vi "Crop Video Time Utility.vi"() -> ()   [LabVIEW 2017]
uses:
  LabVIEW/Controls/Crop Video State.ctl
  LabVIEW/Controls/Frame Grabber Data.ctl
  <vilib>/userdefined/High Color/IMAQdx.ctl
  <vilib>/vision/Image Controls.llb/IMAQ Image.ctl
  <vilib>/vision/Avi.llb/IMAQ AVI2 Refnum.ctl
  LabVIEW/Controls/Rigid Body Info.ctl
  LabVIEW/Controls/Position.ctl
  LabVIEW/Controls/Orientation.ctl
  LabVIEW/Controls/Refnums.ctl
  LabVIEW/Controls/Dimensions.ctl
  LabVIEW/Controls/Room Dimensions.ctl
panel:
  in  "Help":bool
  in  "Codec":u16(ring) items=["Cinepak Codec by Radius", "Intel IYUV codec", "Microsoft Video 1", "FF Video Codec 1 (FFV1) (NI Vision)", "Motion JPEG (NI Vision)", "Y800 Uncompressed Grey Scale (NI Vision)", "YUV 4:2:0 Planar (NI Vision)"]
  out "Number of Playback Frames":i32
  in  "Crop Inside":bool
  in  "Playback Rate":dbl(knob) min=1.0 max=100.0 scale=1.0..100.0
  in  "Crop Outside":bool
  in  "Play":bool
  in  "Frame Slider":cluster{i32, i32, i32}(slide)={9, 173, 93} scale=0.0..1.0
  out "Saving":bool
  in  "Stop":bool
  out "Video path":path
  in  "Load":bool
  out "Frame":T1(plugin-control)
  # "Frame"
  # "of"
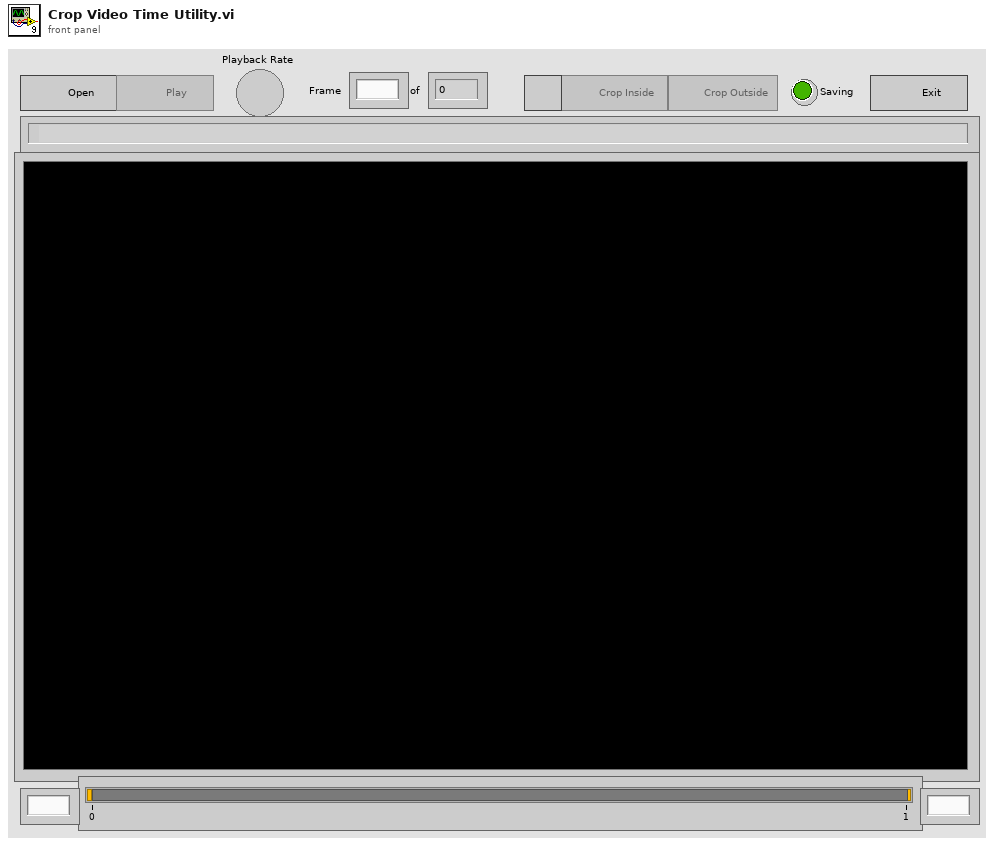
[diagram p1: front panel]
types:
  T1 = typedef "IMAQ Image.ctl" = refnum<image>
  T2 = typedef "Frame Grabber Data.ctl" = cluster{"Camera Session":T3, "Frame":T1, "AVI Refnum":T4, "Codecs":string[], "Frame number":u32, "Tracking File Refnum":refnum<file>, "Tick Count":u32, "Probe Object":refnum<vi>, "Playback Probe Data":dbl[][], "Rigid Body":T5, "Total no frames playback":i32, "Video FPS":dbl, "Camera connected?":bool, "Scene":refnum<vi>, "Cropped Frame":T1, "Tracker FPS":dbl, "Crop ROI":i32[], "Presentation Values":string[], "Elapsed time (ms)":u32, "Camera frames playback":u32, "Refnums":T8, "Dimensions":T9, "Playback Data As Strings":string[][], "Cropped Tracking File Refnum":refnum<file>, "Cropped AVI Refnum":T4, "Header":string[]}
  T3 = typedef "IMAQdx.ctl" = refnum<k21>
  T4 = typedef "IMAQ AVI2 Refnum.ctl" = refnum<k20>
  T5 = typedef "Rigid Body Info.ctl" = cluster{"Position":T6, "Orientation":T7, "Quaternion":cluster{"qx":sgl, "qy":sgl, "qz":sgl, "qw":sgl}, "Tracked?":bool}
  T6 = typedef "Position.ctl" = cluster{"x (mm)":sgl, "y (mm)":sgl, "z (mm)":sgl}
  T7 = typedef "Orientation.ctl" = cluster{"Pitch (rad)":sgl, "Yaw (rad)":sgl, "Roll (rad)":sgl}
  T8 = typedef "Refnums.ctl" = cluster{"Live Refnum":refnum<vi>, "Record Refnum":refnum<vi>, "Recording Settings Refnum":refnum<vi>, "Playback Refnum":refnum<vi>, "Frame Slider Refnum":refnum<vi>, "Pause Refnum":refnum<vi>, "Home Refnum":refnum<vi>, "Crop Refnum":refnum<vi>, "Clear Crop Refnum":refnum<vi>, "stop refnum":refnum<vi>, "Playback Rate Refnum":refnum<vi>, "Operator Settings Refnums":refnum<vi>, "Presentation Refnum":refnum<vi>, "Gestation Refnum":refnum<vi>, "Connection Settings Refnum":refnum<vi>, "Crop Time Frame Slider Refnum":refnum<vi>}
  T9 = typedef "Dimensions.ctl" = cluster{"Probe Dimensions":cluster{"Probe Width":sgl, "Probe Depth":sgl, "Probe Height":sgl}, "Room Dimensions":T10}
  T10 = typedef "Room Dimensions.ctl" = cluster{"Room Width":dbl, "Room Depth":dbl, "Room Height":dbl}
  T11 = typedef "Crop Video State.ctl" = enum16{"Init", "Wait", "Load", "Playback Frame", "Save", "Close", "Crop Inside", "Crop Outside", "Error Handling", "Shutdown"}
  T12 = enum8{"Enabled", "Disabled", "Disabled and Grayed Out"}
  T13 = typedef "Image Type" = u32
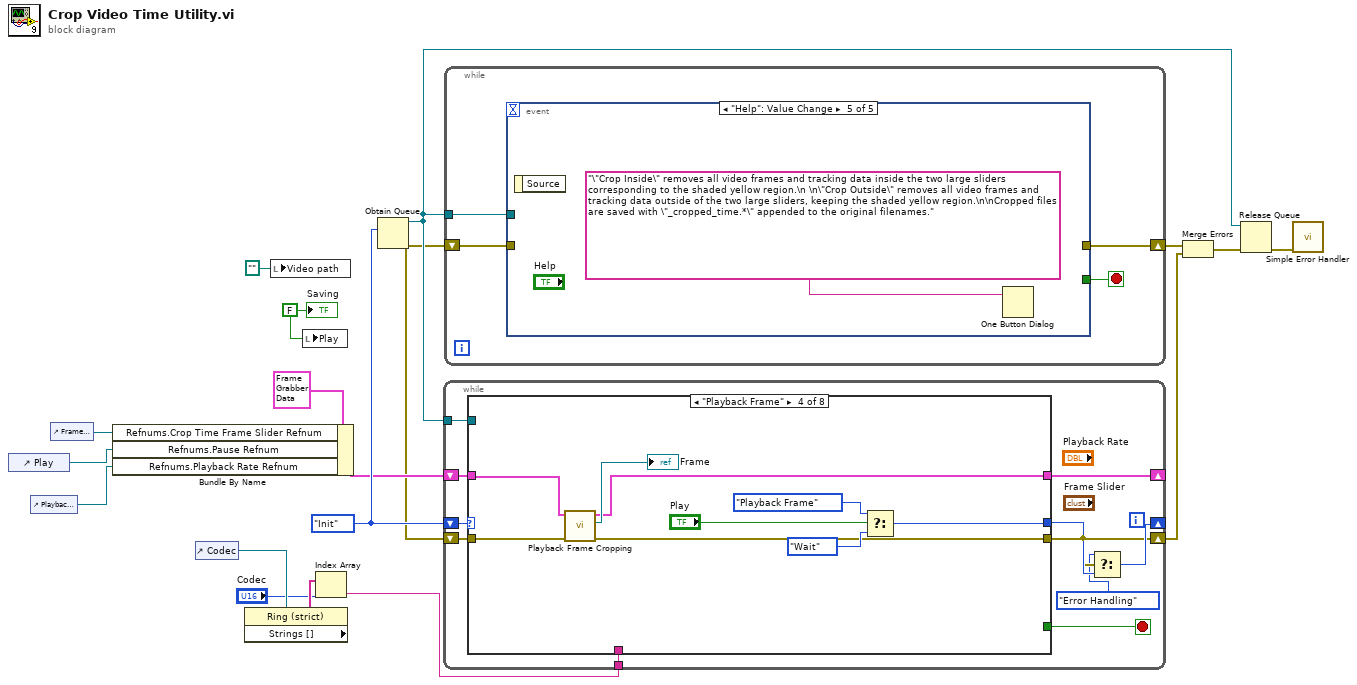
[diagram p0: block diagram]
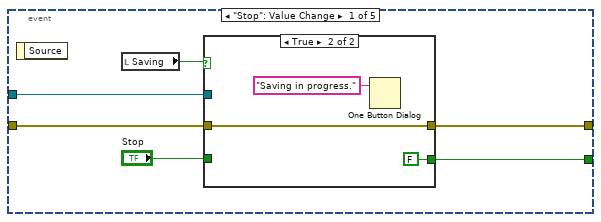
[diagram p2: hidden frame]
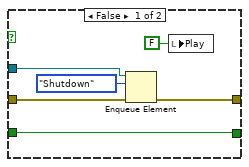
[diagram p3: hidden frame]
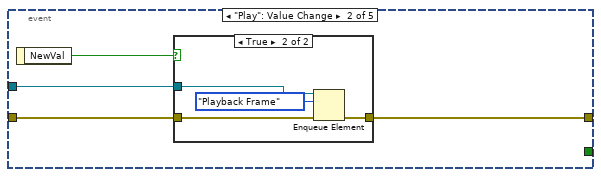
[diagram p4: hidden frame]
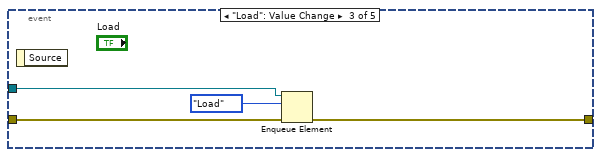
[diagram p6: hidden frame]
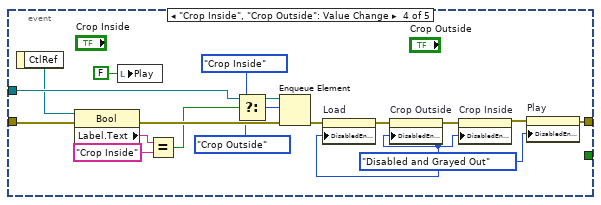
[diagram p7: hidden frame]
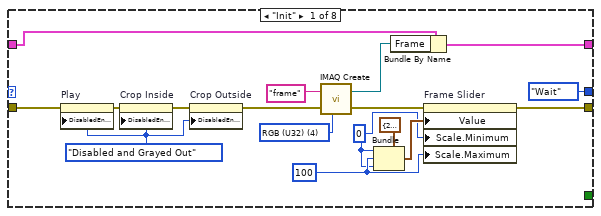
[diagram p8: hidden frame]
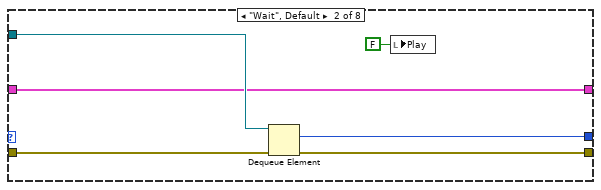
[diagram p9: hidden frame]
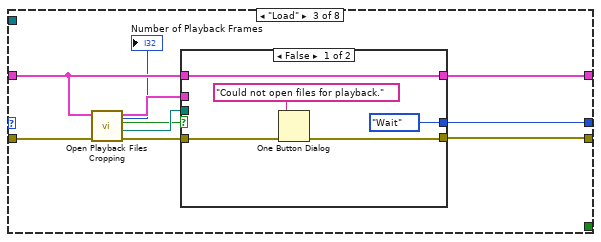
[diagram p10: hidden frame]
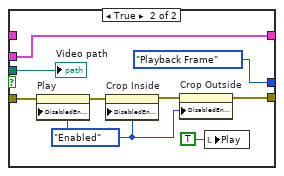
[diagram p11: hidden frame]
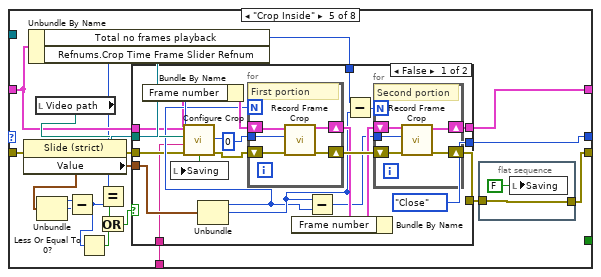
[diagram p12: hidden frame]
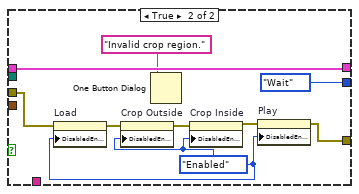
[diagram p13: hidden frame]
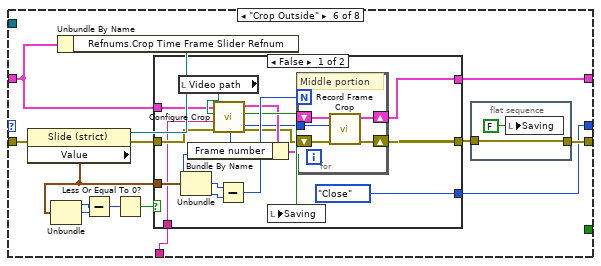
[diagram p14: hidden frame]
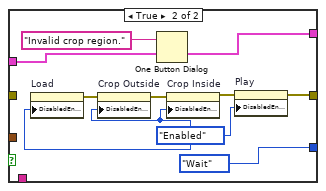
[diagram p15: hidden frame]
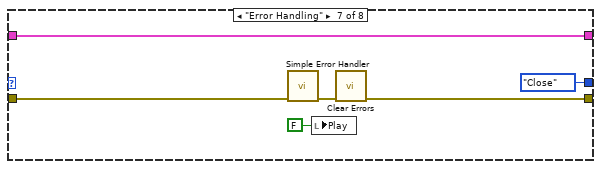
[diagram p16: hidden frame]
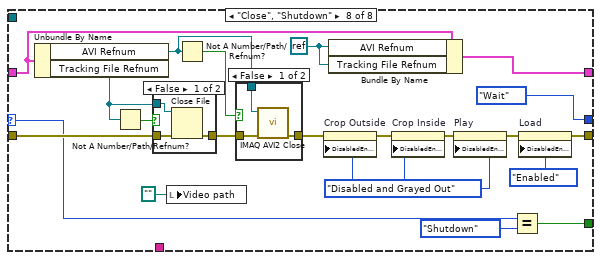
[diagram p17: hidden frame]
diagram:
  w18 = Crop_Video_State."Init" ("State")
  w6 = FALSE ("Saving")
  n1 = control-ref of="Play"() -> (w13:refnum<vi>)
  n2 = control-ref of="Playback Rate"() -> (w12:refnum<vi>)
  n3 = control-ref of="Frame Slider"() -> (w5:refnum<vi>)
  n4 = Bundle By Name(cluster=T2 {"Camera Session"="", "Frame"=refnum, "AVI Refnum"=refnum, "Codecs"=[], "Frame number"=0, "Tracking File Refnum"=refnum, "Tick Count"=0, "Probe Object"=refnum, "Playback Probe Data"=[], "Rigid Body"={"Position"={"x (mm)"=0.0, "y (mm)"=0.0, "z (mm)"=0.0}, "Orientation"={"Pitch (rad)"=0.0, "Yaw (rad)"=0.0, "Roll (rad)"=0.0}, "Quaternion"={"qx"=0.0, "qy"=0.0, "qz"=0.0, "qw"=0.0}, "Tracked?"=FALSE}, "Total no frames playback"=0, "Video FPS"=0.0, "Camera connected?"=FALSE, "Scene"=refnum, "Cropped Frame"=refnum, "Tracker FPS"=0.0, "Crop ROI"=[], "Presentation Values"=[], "Elapsed time (ms)"=0, "Camera frames playback"=0, "Refnums"={"Live Refnum"=refnum, "Record Refnum"=refnum, "Recording Settings Refnum"=refnum, "Playback Refnum"=refnum, "Frame Slider Refnum"=refnum, "Pause Refnum"=refnum, "Home Refnum"=refnum, "Crop Refnum"=refnum, "Clear Crop Refnum"=refnum, "stop refnum"=refnum, "Playback Rate Refnum"=refnum, "Operator Settings Refnums"=refnum, "Presentation Refnum"=refnum, "Gestation Refnum"=refnum, "Connection Settings Refnum"=refnum, "Crop Time Frame Slider Refnum"=refnum}, "Dimensions"={"Probe Dimensions"={"Probe Width"=0.0, "Probe Depth"=1.0, "Probe Height"=0.0}, "Room Dimensions"={"Room Width"=0.0, "Room Depth"=0.0, "Room Height"=0.0}}, "Playback Data As Strings"=[], "Cropped Tracking File Refnum"=refnum, "Cropped AVI Refnum"=refnum, "Header"=[]} ("Frame Grabber Data 2"), "Refnums.Crop Time Frame Slider Refnum"=w5, "Refnums.Pause Refnum"=w13, "Refnums.Playback Rate Refnum"=w12) -> (w9:T2)
  n5 = control-ref of="Codec"() -> (w4:refnum<vi>)
  n6 = property class="Ring (strict)"(reference=w4) -> ("Strings []"=w3:string[])  [unwired: 1 in, 2 out]
  n7 = local write "Video path"(path "") -> ()
  n8 = local write "Play"(w6) -> ()
  n9 = Index Array(array=w3, index="Codec") -> (element=w1:string)
  n10 = Obtain Queue(element data type=w18) -> (queue out=w14:refnum<queue>, error out=w8:errorcluster)  [unwired: 4 in, 1 out]
  n11 = while {
    shift-right: [w24] -> _
    shift-left: w9 -> [w25]
    tunnel: w14 -> [w27]
    shift-right: [w21] -> w16
    shift-left: w8 -> [w26]
    shift-right: [w22] -> _
    shift-left: w18 -> [w29]
    tunnel: w1 -> [w19]
    stop <- w28 stop-if-true
    n12 = case shown="\"Playback Frame\"" w29 {
      selector: w29 -> [_ _ _ _ _ _ _ w201]
      tunnel: [_ _ _ _ _ _ _ w199] -> w28
      tunnel: w27 -> [_ w52 _ _ _ _ _ _]
      tunnel: w26 -> [w36 w51 w62 w79 w97 w153 w194 w214]
      tunnel: [w37 w50 w55 w77 w98 w155 w192 w196] -> w21
      tunnel: [Crop_Video_State."Wait" ("State") w49 w54 w82 w94 w151 Crop_Video_State."Close" ("State") Crop_Video_State."Wait" ("State")] -> w23
      tunnel: w25 -> [w44 w48 w57 w80 w96 w154 w189 w207]
      tunnel: [w41 w48 w59 w78 w102 w157 w189 w203] -> w24
      tunnel: w19 -> [_ _ _ _ w85 w145 _ _]
      frame "Init" {
        w32 = T12."Disabled and Grayed Out" ("Disabled")
        w31 = u32 100 ("Frame")
        w30 = u32 0 ("Min")
        w45 = T13 4 items=["Grayscale (U8)", "Grayscale (I16)", "Grayscale (SGL)", "Complex (CSG)", "RGB (U32)", "HSL (U32)", "RGB (U64)", "Grayscale (U16)"] ("Image Type")
        n13 = property on="Play" class="Bool (strict)"(error in=w36, "DisabledEnum"=w32) -> (error out=w33:errorcluster)  [unwired: 1 in, 1 out]
        n14 = property on="Crop Inside" class="Bool"(error in=w33, "DisabledEnum"=w32) -> (error out=w34:errorcluster)  [unwired: 1 in, 1 out]
        n15 = property on="Crop Outside" class="Bool"(error in=w34, "DisabledEnum"=w32) -> (error out=w35:errorcluster)  [unwired: 1 in, 1 out]
        n16 = call "IMAQ Create"("Image Name"="frame", "Image Type"=w45, "error in (no error)"=w35) -> ("New Image"=w43:T1, "error out"=w38:errorcluster)  [unwired: 2 in]
        n17 = Bundle(cluster=cluster{"Min":u32, "Max":u32, "Frame":u32} {"Min"=24, "Max"=167, "Frame"=33} ("Frame Slider"), "Min"=w30, "Max"=w31, "Frame"=w30) -> (w40:cluster{"Min":u32, "Max":u32, "Frame":u32})
        n18 = Bundle By Name(cluster=w44, "Frame"=w43) -> (w41:T2)
        n19 = property on="Frame Slider" class="Slide (strict)"(error in=w38, "Value"=w40, "Scale.Minimum"=w30, "Scale.Maximum"=w31) -> (error out=w37:errorcluster)  [unwired: 1 in, 1 out]
      }
      frame "Wait", Default {
        n20 = Dequeue Element(queue=w52, error in (no error)=w51) -> (element=w49:T11, error out=w50:errorcluster)  [unwired: 1 in, 2 out]
        n21 = local write "Play"(FALSE) -> ()
      }
      frame "Load" {
        n22 = call "Open Playback Files Cropping.vi"("error in (no error)"=w62, "Frame Grabber Data In"=w57) -> ("error out"=w60:errorcluster, "Playback Video"=w61:path, "both exist and open?"=w56:bool, "Frame Grabber Data Out"=w58:T2, "Number of Playback Frames"=→"Number of Playback Frames":i32)  [unwired: 4 in, 1 out]
        n23 = case shown="False" w56 {
          tunnel: w61 -> [_ w75]
          tunnel: w60 -> [w65 w74]
          tunnel: [w66 w73] -> w59
          tunnel: w58 -> [_ w73]
          tunnel: w57 -> [w66 _]
          tunnel: [w65 w72] -> w55
          tunnel: [Crop_Video_State."Wait" ("State") Crop_Video_State."Playback Frame" ("State")] -> w54
          frame False {
            n24 = One Button Dialog(message="Could not open files for playback.") -> ()  [unwired: 1 in, 1 out]
          }
          frame True {
            w69 = T12."Enabled" ("Disabled")
            n25 = property on="Play" class="Bool (strict)"(error in=w74, "DisabledEnum"=w69) -> (error out=w70:errorcluster)  [unwired: 1 in, 1 out]
            n26 = property on="Crop Inside" class="Bool"(error in=w70, "DisabledEnum"=w69) -> (error out=w71:errorcluster)  [unwired: 1 in, 1 out]
            n27 = property on="Crop Outside" class="Bool"(error in=w71, "DisabledEnum"=w69) -> (error out=w72:errorcluster)  [unwired: 1 in, 1 out]
            n28 = local write "Play"(TRUE ("Play")) -> ()
            "Video path" <- w75
          }
        }
      }
      frame "Playback Frame" {
        n29 = call "Playback Frame Cropping.vi"("error in (no error)"=w79, "Frame Grabber Data in"=w80) -> ("error out"=w77:errorcluster, "Image"=→"Frame":T1, "Frame Grabber Data out"=w78:T2)  [unwired: 5 in, 2 out]
        n30 = Select(t=Crop_Video_State."Playback Frame" ("State"), s="Play", f=Crop_Video_State."Wait" ("State")) -> (s? t:f=w82:T11)
      }
      frame "Crop Inside" {
        n31 = Unbundle By Name(w96) -> ("Total no frames playback"=w91:i32, "Refnums.Crop Time Frame Slider Refnum"=w101:refnum<vi>)
        n32 = property class="Slide (strict)"(reference=w101, error in=w97) -> (error out=w95:errorcluster, "Value"=w93:cluster{i32, i32, i32})  [unwired: 1 out]
        n33 = local read "Video path"() -> (w100:path)
        n34 = Unbundle(w93) -> (w90:i32, w89:i32)  [unwired: 1 out]
        n35 = Subtract(x=w89, y=w90) -> (x-y=w86:i32)
        n36 = Less Or Equal To 0?(x=w86) -> (x <= 0?=w87:bool)
        n37 = Equal?(x=w91, y=w86) -> (x = y?=w92:bool)
        n38 = Or(x=w92, y=w87) -> (x .or. y?=w88:bool)
        n39 = case shown="False" w88 {
          tunnel: [w122 w142] -> w102
          tunnel: w93 -> [w121 _]
          tunnel: w100 -> [w118 _]
          tunnel: [w117 w134] -> w99
          tunnel: w91 -> [w112 _]
          tunnel: w96 -> [w108 w142]
          tunnel: w95 -> [w106 w136]
          tunnel: [Crop_Video_State."Close" ("State") Crop_Video_State."Wait" ("State")] -> w94
          tunnel: w85 -> [w103 _]
          frame False {
            w115 = u32 0 ("Starting frame number")
            n40 = call "Configure Crop.vi"("error in (no error)"=w106, "Codec"=w103, "Video file path"=w118, "Frame Grabber Data In"=w108) -> ("error out"=w105:errorcluster, "Saving?"=w119:bool, "Frame Grabber Data Out"=w107:T2)  [unwired: 5 in]
            n41 = Bundle By Name(cluster=w107, "Frame number"=w115) -> (w116:T2)
            n42 = local write "Saving"(w119) -> ()
            n43 = Unbundle(w121) -> (w110:i32, w111:i32)  [unwired: 1 out]
            n44 = for {
              N: w110 -> [_]
              shift-right: [w132] -> w123
              shift-left: w105 -> [w133]
              shift-right: [w130] -> w114
              shift-left: w116 -> [w131]
              tunnel: w115 -> [w129]
              # "First portion"
              n45 = call "Record Frame Crop.vi"("error in (no error)"=w133, "Starting frame number"=w129, "Frame Grabber Data In in"=w131) -> ("error out"=w132:errorcluster, "Frame Grabber Data out"=w130:T2)  [unwired: 7 in]
            }
            n46 = Bundle By Name(cluster=w114, "Frame number"=w111) -> (w113:T2)
            n47 = Subtract(x=w111, y=w110) -> (x-y=w109:i32)
            n48 = Subtract(x=w112, y=w111) -> (x-y=w120:i32)
            n49 = for {
              N: w120 -> [_]
              shift-right: [w127] -> w117
              shift-left: w123 -> [w128]
              shift-right: [w125] -> w122
              shift-left: w113 -> [w126]
              tunnel: w109 -> [w124]
              # "Second portion"
              n50 = call "Record Frame Crop.vi"("error in (no error)"=w128, "Starting frame number"=w124, "Frame Grabber Data In in"=w126) -> ("error out"=w127:errorcluster, "Frame Grabber Data out"=w125:T2)  [unwired: 7 in]
            }
          }
          frame True {
            w135 = T12."Enabled" ("Disabled")
            n51 = property on="Load" class="Bool"(error in=w136, "DisabledEnum"=w135) -> (error out=w139:errorcluster)  [unwired: 1 in, 1 out]
            n52 = property on="Crop Outside" class="Bool"(error in=w139, "DisabledEnum"=w135) -> (error out=w138:errorcluster)  [unwired: 1 in, 1 out]
            n53 = One Button Dialog(message="Invalid crop region.") -> ()  [unwired: 1 in, 1 out]
            n54 = property on="Crop Inside" class="Bool"(error in=w138, "DisabledEnum"=w135) -> (error out=w137:errorcluster)  [unwired: 1 in, 1 out]
            n55 = property on="Play" class="Bool (strict)"(error in=w137, "DisabledEnum"=w135) -> (error out=w134:errorcluster)  [unwired: 1 in, 1 out]
          }
        }
        n56 = flat-sequence {
          tunnel: w99 -> [w143]
          tunnel: [w143] -> _
          tunnel: [w143] -> w98
          frame #0 {
            n57 = local write "Saving"(FALSE) -> ()
          }
        }
      }
      frame "Crop Outside" {
        n58 = Unbundle By Name(w154) -> ("Refnums.Crop Time Frame Slider Refnum"=w158:refnum<vi>)
        n59 = property class="Slide (strict)"(reference=w158, error in=w153) -> (error out=w152:errorcluster, "Value"=w150:cluster{i32, i32, i32})  [unwired: 1 out]
        n60 = Unbundle(w150) -> (w148:i32, w149:i32)  [unwired: 1 out]
        n61 = Subtract(x=w149, y=w148) -> (x-y=w147:i32)
        n62 = Less Or Equal To 0?(x=w147) -> (x <= 0?=w146:bool)
        n63 = case shown="False" w146 {
          tunnel: w150 -> [w173 _]
          tunnel: [w170 w186] -> w157
          tunnel: [w169 w179] -> w156
          tunnel: w154 -> [w163 w186]
          tunnel: w152 -> [w162 _]
          tunnel: [Crop_Video_State."Close" ("State") Crop_Video_State."Wait" ("State")] -> w151
          tunnel: w145 -> [w159 _]
          frame False {
            n64 = local read "Video path"() -> (w167:path)
            n65 = Unbundle(w173) -> (w164:i32, w172:i32)  [unwired: 1 out]
            n66 = call "Configure Crop.vi"("error in (no error)"=w162, "Codec"=w159, "Video file path"=w167, "Frame Grabber Data In"=w163) -> ("error out"=w161:errorcluster, "Saving?"=w168:bool, "Frame Grabber Data Out"=w166:T2)  [unwired: 5 in]
            n67 = Bundle By Name(cluster=w166, "Frame number"=w164) -> (w165:T2)
            n68 = Subtract(x=w172, y=w164) -> (x-y=w171:i32)
            n69 = local write "Saving"(w168) -> ()
            n70 = for {
              N: w171 -> [_]
              shift-right: [w177] -> w169
              shift-left: w161 -> [w178]
              tunnel: w164 -> [w176]
              shift-right: [w175] -> w170
              shift-left: w165 -> [w174]
              # "Middle portion"
              n71 = call "Record Frame Crop.vi"("error in (no error)"=w178, "Starting frame number"=w176, "Frame Grabber Data In in"=w174) -> ("error out"=w177:errorcluster, "Frame Grabber Data out"=w175:T2)  [unwired: 7 in]
            }
          }
          frame True {
            w180 = T12."Enabled" ("Disabled")
            n72 = property on="Load" class="Bool"("DisabledEnum"=w180) -> (error out=w183:errorcluster)  [unwired: 2 in, 1 out]
            n73 = property on="Crop Outside" class="Bool"(error in=w183, "DisabledEnum"=w180) -> (error out=w182:errorcluster)  [unwired: 1 in, 1 out]
            n74 = One Button Dialog(message="Invalid crop region.") -> ()  [unwired: 1 in, 1 out]
            n75 = property on="Crop Inside" class="Bool"(error in=w182, "DisabledEnum"=w180) -> (error out=w181:errorcluster)  [unwired: 1 in, 1 out]
            n76 = property on="Play" class="Bool (strict)"(error in=w181, "DisabledEnum"=w180) -> (error out=w179:errorcluster)  [unwired: 1 in, 1 out]
          }
        }
        n77 = flat-sequence {
          tunnel: w156 -> [w188]
          tunnel: [w188] -> w155
          frame #0 {
            n78 = local write "Saving"(FALSE) -> ()
          }
        }
      }
      frame "Error Handling" {
        n79 = call <vilib>:"Simple Error Handler.vi"("error in (no error)"=w194) -> ("error out"=w193:errorcluster)  [unwired: 4 in, 4 out]
        n80 = local write "Play"(FALSE ("Play")) -> ()
        n81 = call <vilib>:"Clear Errors.vi"("error in (no error)"=w193) -> ("error out"=w192:errorcluster)  [unwired: 5 in, 1 out]
      }
      frame "Close", "Shutdown" {
        w202 = refnum<k0> refnum
        w205 = T12."Disabled and Grayed Out" ("Disabled")
        n82 = Unbundle By Name(w207) -> ("AVI Refnum"=w209:T4, "Tracking File Refnum"=w212:refnum<file>)
        n83 = Not A Number/Path/Refnum?(number/path/refnum=w212) -> (NaN/Path/Refnum?=w213:bool)
        n84 = case shown="False" w213 {
          tunnel: w214 -> [w222 w223]
          tunnel: [w221 w223] -> w211
          tunnel: w212 -> [w220 _]
          frame False {
            n85 = Close File(refnum=w220, error in=w222) -> (error out=w221:errorcluster)  [unwired: 1 out]
          }
          frame True {
          }
        }
        n86 = local write "Video path"(path "") -> ()
        n87 = Not A Number/Path/Refnum?(number/path/refnum=w209) -> (NaN/Path/Refnum?=w208:bool)
        n88 = case shown="False" w208 {
          tunnel: w211 -> [w218 w219]
          tunnel: [w217 w219] -> w210
          tunnel: w209 -> [w216 _]
          frame False {
            n89 = call "IMAQ AVI2 Close"("error in (no error)"=w218, "AVI Refnum"=w216) -> ("error out"=w217:errorcluster)  [unwired: 9 in]
          }
          frame True {
          }
        }
        n90 = property on="Crop Outside" class="Bool"(error in=w210, "DisabledEnum"=w205) -> (error out=w206:errorcluster)  [unwired: 1 in, 1 out]
        n91 = Bundle By Name(cluster=w207, "AVI Refnum"=w202, "Tracking File Refnum"=w202) -> (w203:T2)
        n92 = property on="Crop Inside" class="Bool"(error in=w206, "DisabledEnum"=w205) -> (error out=w204:errorcluster)  [unwired: 1 in, 1 out]
        n93 = property on="Play" class="Bool (strict)"(error in=w204, "DisabledEnum"=w205) -> (error out=w197:errorcluster)  [unwired: 1 in, 1 out]
        n94 = Equal?(x=w201, y=Crop_Video_State."Shutdown") -> (x = y?=w199:bool)
        n95 = property on="Load" class="Bool"(error in=w197, "DisabledEnum"=T12."Enabled" ("Disabled")) -> (error out=w196:errorcluster)  [unwired: 1 in, 1 out]
      }
    }
    n96 = Select(t=Crop_Video_State."Error Handling", s=w21, f=w23) -> (s? t:f=w22:T11)
  }
  n97 = while {
    tunnel: w14 -> [w226]
    shift-right: [w224] -> w17
    shift-left: w8 -> [w225]
    stop <- w227 stop-if-true
    n98 = event shown="[4] \"Help\": Value Change" {
      selector: _ -> [_ _ _ _ _]
      dyn-events: _ -> [_ _ _ _ _]
      timeout: _ -> [_ _ _ _ _]
      tunnel: [w231 _ _ _ _] -> w227
      tunnel: w226 -> [w230 w244 w253 w272 _]
      tunnel: w225 -> [w229 w246 w255 w270 _]
      tunnel: [w228 w245 w254 w259 _] -> w224
      event "Stop": Value Change {
        n99 = event-data() -> ()  [unwired: 1 in, 1 out]
        n100 = local read "Saving"() -> (w233:bool)
        n101 = case shown="True" w233 {
          tunnel: "Stop" -> [w239 _]
          tunnel: [w239 FALSE] -> w231
          tunnel: w230 -> [w238 _]
          tunnel: w229 -> [w237 w240]
          tunnel: [w236 w240] -> w228
          frame False {
            n102 = Enqueue Element(queue=w238, element=Crop_Video_State."Shutdown", error in (no error)=w237) -> (error out=w236:errorcluster)  [unwired: 1 in, 2 out]
            n103 = local write "Play"(FALSE ("Play")) -> ()
          }
          frame True {
            n104 = One Button Dialog(message="Saving in progress.") -> ()  [unwired: 1 in, 1 out]
          }
        }
      }
      event "Play": Value Change {
        n105 = event-data() -> ("NewVal"=w243:bool)  [unwired: 1 in]
        n106 = case shown="True" w243 {
          tunnel: w246 -> [w247 w251]
          tunnel: [w247 w250] -> w245
          tunnel: w244 -> [_ w249]
          frame False {
          }
          frame True {
            n107 = Enqueue Element(queue=w249, element=Crop_Video_State."Playback Frame", error in (no error)=w251) -> (error out=w250:errorcluster)  [unwired: 1 in, 2 out]
          }
        }
      }
      event "Load": Value Change {
        n108 = event-data() -> ()  [unwired: 1 in, 1 out]
        n109 = Enqueue Element(queue=w253, element=Crop_Video_State."Load", error in (no error)=w255) -> (error out=w254:errorcluster)  [unwired: 1 in, 2 out]
      }
      event "Crop Inside", "Crop Outside": Value Change {
        w256 = T12."Disabled and Grayed Out" ("Disabled")
        n110 = event-data() -> ("CtlRef"=w268:refnum<vi>)  [unwired: 1 in]
        n111 = property class="Bool"(reference=w268, error in=w270) -> (error out=w269:errorcluster, "Label.Text"=w267:string)  [unwired: 1 out]
        n112 = local write "Play"(FALSE ("Play")) -> ()
        n113 = Equal?(x=w267, y="Crop Inside") -> (x = y?=w264:bool)
        n114 = Select(t=Crop_Video_State."Crop Inside" ("element"), s=w264, f=Crop_Video_State."Crop Outside") -> (s? t:f=w265:T11)
        n115 = Enqueue Element(queue=w272, element=w265, error in (no error)=w269) -> (error out=w257:errorcluster)  [unwired: 1 in, 2 out]
        n116 = property on="Load" class="Bool"(error in=w257, "DisabledEnum"=w256) -> (error out=w258:errorcluster)  [unwired: 1 in, 1 out]
        n117 = property on="Crop Outside" class="Bool"(error in=w258, "DisabledEnum"=w256) -> (error out=w260:errorcluster)  [unwired: 1 in, 1 out]
        n118 = property on="Crop Inside" class="Bool"(error in=w260, "DisabledEnum"=w256) -> (error out=w261:errorcluster)  [unwired: 1 in, 1 out]
        n119 = property on="Play" class="Bool (strict)"(error in=w261, "DisabledEnum"=w256) -> (error out=w259:errorcluster)  [unwired: 1 in, 1 out]
      }
      event "Help": Value Change {
        n120 = event-data() -> ()  [unwired: 1 in, 1 out]
        n121 = One Button Dialog(message="\"Crop Inside\" removes all video frames and tracking data inside the two large sliders corresponding to the shaded yellow region.\n \n\"Crop Outside\" removes all video frames and tracking data outside of the two large sliders, keeping the shaded yellow region.\n\nCropped files are saved with \"_cropped_time.*\" appended to the original filenames.") -> ()  [unwired: 1 in, 1 out]
      }
    }
  }
  n122 = Merge Errors(w17, w16) -> (w15:errorcluster)
  n123 = Release Queue(queue=w14, error in (no error)=w15) -> (error out=w10:errorcluster)  [unwired: 1 in, 2 out]
  n124 = call <vilib>:"Simple Error Handler.vi"("error in (no error)"=w10) -> ()  [unwired: 4 in, 5 out]
  "Saving" <- w6
